vi "Get Limit Test Enabled State.vi"(0 "VISA resource name":refnum<visa-resource-name>, 5 "Limit Test Number (2)":u16=2, 7 "Function (0: Volts)":u16(ring) items=["Volts", "Current", "Resistance", "Digitize Voltage", "Digitize Current"], 11 "error in (no error)":errorcluster) -> (4 "VISA resource name out":refnum<visa-resource-name>, 6 "Limit Test Enabled?":bool, 15 "error out":errorcluster)   [LabVIEW 2021, in "Keithley 2450.lvlib"]
doc: "Gets the state of the selected limit test."
uses:
  <instrlib>/Keithley 2450/Keithley 2450.lvlib
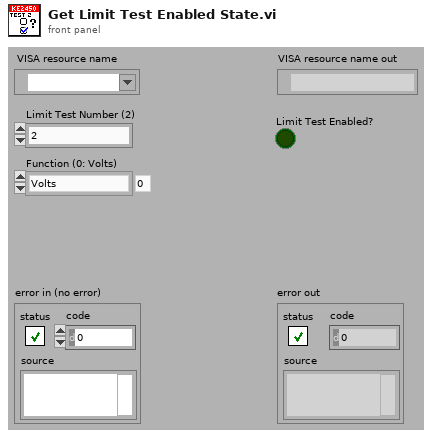
[diagram p1: front panel]
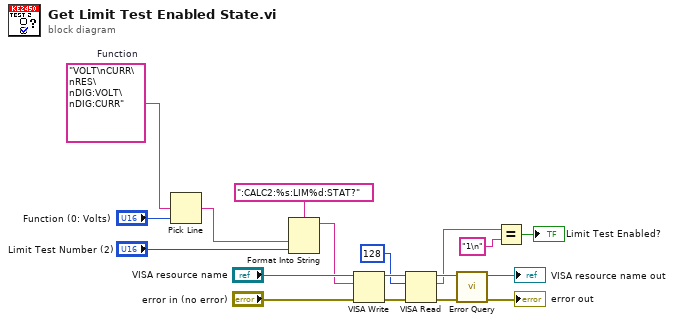
[diagram p0: block diagram]
diagram:
  w12 = "VOLT\nCURR\nRES\nDIG:VOLT\nDIG:CURR"  # Function
  n1 = Pick Line(multi-line string=w12, line index="Function (0: Volts)") -> (output string=w10:string)  [unwired: 1 out]
  n2 = Format Into String(format string=":CALC2:%s:LIM%d:STAT?", w10, "Limit Test Number (2)") -> (resulting string=w13:string)  [unwired: 2 in, 1 out]
  n3 = VISA Write(VISA resource name="VISA resource name", write buffer=w13, error in (no error)="error in (no error)") -> (VISA resource name out=w6:refnum<visa-resource-name>, error out=w8:errorcluster)  [unwired: 1 out]
  n4 = VISA Read(VISA resource name=w6, byte count=u32 128, error in (no error)=w8) -> (VISA resource name out=w5:refnum<visa-resource-name>, read buffer=w1:string, error out=w7:errorcluster)  [unwired: 1 out]
  n5 = call <instrlib>:"Error Query.vi"("error in (no error)"=w7, "VISA resource name"=w5) -> ("error out"=→"error out":errorcluster, "VISA resource name out"=→"VISA resource name out":refnum<visa-resource-name>)  [unwired: 8 out]
  n6 = Equal?(x=w1, y="1\n") -> (x = y?=→"Limit Test Enabled?":bool)
